vi "buildITaskMethodPath.vi"(1 "methodName":string) -> (0 "ITaskMethodPath":path)   [LabVIEW 2023]
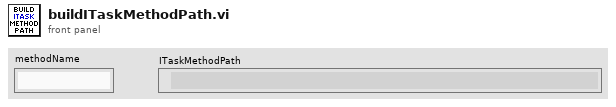
[diagram p1: front panel]
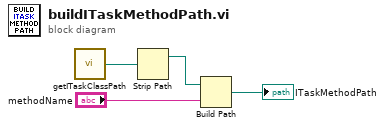
[diagram p0: block diagram]
diagram:
  n1 = call "getITaskClassPath.vi"() -> ("ITaskClassPath"=w4:path)
  n2 = Strip Path(path=w4) -> (stripped path=w3:path)  [unwired: 1 out]
  n3 = Build Path(base path=w3, name or relative path="methodName") -> (appended path=→"ITaskMethodPath":path)
